vi "Find Scan Engine Custom Device.vi"(8 "error in":errorcluster, 11 "target in":refnum<k24>) -> (0 "error out":errorcluster, 2 "scan engine custom device ref":T1 format="%.0x", 3 "target out":refnum<k24>, 4 "found":bool)   [LabVIEW 2020, in "Scan Engine Scripting.lvlib"]
doc: "Returns the Scan Engine and EtherCAT custom device found in the specified target."
uses:
  Scan Engine Scripting.lvlib
  NationalInstruments.VeriStand.SystemDefinitionAPI
  <vilib>/NI VeriStand/Custom Device API/Custom Device Item Ref.ctl
  Scan Engine Dependencies.llb/Scan Engine GUIDs.vi
  Utility/Ref Constants.vi
  Scan Engine Dependencies.llb/Scan Engine Custom Device.lvlib
  <vilib>/NI VeriStand/Custom Device API/Custom Device API.lvlib
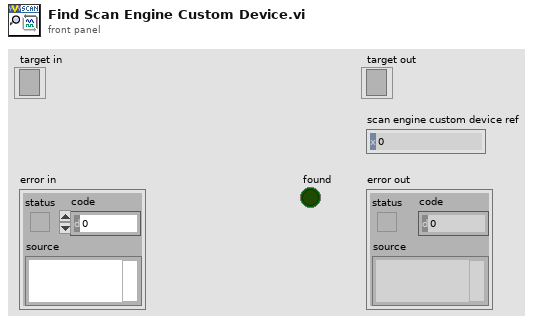
[diagram p1: front panel]
types:
  T1 = typedef "Custom Device API.lvlib/Custom Device Item Ref.ctl" = u64
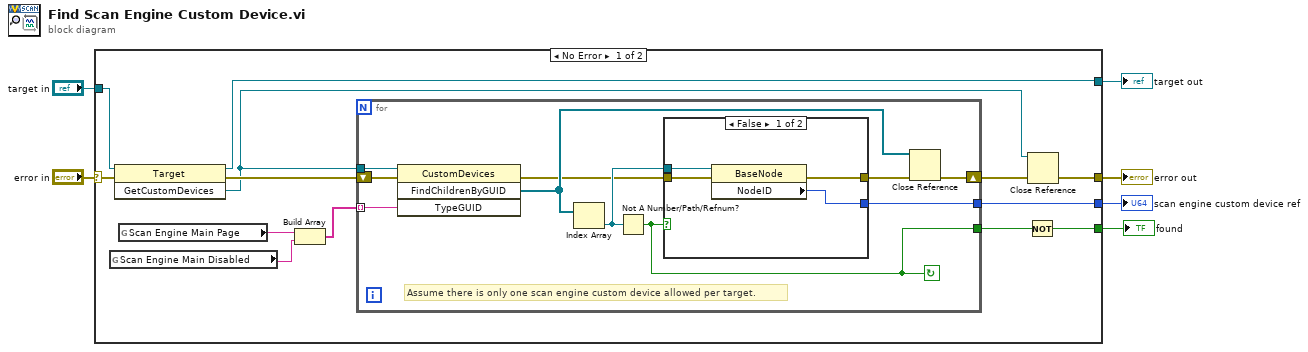
[diagram p0: block diagram]
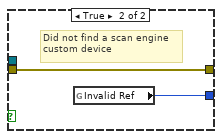
[diagram p2: hidden frame]
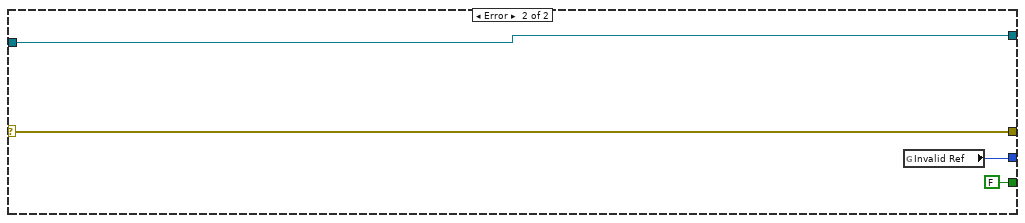
[diagram p3: hidden frame]
diagram:
  n1 = case shown="No Error" "error in" {
    selector: "error in" -> [w19 w39]
    tunnel: [w8 w39] -> w6
    tunnel: "target in" -> [w18 w38]
    tunnel: [w16 w38] -> w3
    tunnel: [w15 w36] -> w2
    tunnel: [w10 FALSE] -> w1
    frame No Error {
      n2 = global read "Scan Engine GUIDs.vi" "Scan Engine Main Disabled"() -> (w13:string)
      n3 = invoke class="Target" method="GetCustomDevices"(reference=w18, error in=w19) -> (reference out=w16:refnum<k24>, error out=w17:errorcluster, "GetCustomDevices"=w7:refnum<k24>)  [unwired: 1 in]
      n4 = global read "Scan Engine GUIDs.vi" "Scan Engine Main Page"() -> (w14:string)
      n5 = Build Array(w14, w13) -> (w12:string[])
      n6 = for {
        tunnel: w7 -> [w28]
        tunnel: [w27] -> w15
        shift-right: [w26] -> w9
        shift-left: w17 -> [w29]
        tunnel: w12 -> [w23] mode=indexing
        tunnel: [w21] -> w11
        stop <- w21 continue-if-true
        # "Assume there is only one scan engine custom device allowed per target."
        n7 = invoke class="CustomDevices" method="FindChildrenByGUID"(reference=w28, error in=w29, "TypeGUID"=w23) -> (error out=w20:errorcluster, "FindChildrenByGUID"=w24:refnum<k24>[])  [unwired: 1 in, 2 out]
        n8 = Index Array(array=w24) -> (element=w22:refnum<k24>)  [unwired: 1 in]
        n9 = Not A Number/Path/Refnum?(number/path/refnum=w22) -> (NaN/Path/Refnum?=w21:bool)
        n10 = case shown="False" w21 {
          tunnel: [w30 w35] -> w25
          tunnel: w20 -> [w31 w35]
          tunnel: w22 -> [w33 _]
          tunnel: [w32 w34] -> w27
          frame False {
            n11 = property class="BaseNode"(reference=w33, error in=w31) -> (error out=w30:errorcluster, "NodeID"=w32:u64)  [unwired: 1 out]
          }
          frame True {
            # "Did not find a scan engine custom device"
            n12 = global read "Ref Constants.vi" "Invalid Ref"() -> (w34:T1)
          }
        }
        n13 = Close Reference(reference=w24, error in (no error)=w25) -> (error out=w26:errorcluster)
      }
      n14 = Not(x=w11) -> (.not. x?=w10:bool)
      n15 = Close Reference(reference=w7, error in (no error)=w9) -> (error out=w8:errorcluster)
    }
    frame Error {
      n16 = global read "Ref Constants.vi" "Invalid Ref"() -> (w36:T1)
    }
  }
  "target out" <- w3
  "error out" <- w6
  "scan engine custom device ref" <- w2
  "found" <- w1
